vi "z2.vi"() -> ()   [LabVIEW 2023]
uses:
  Kontrola.ctl
panel:
  in  "10D":bool
  in  "5D":bool
  in  "stop 2":bool
  out "Numeric 3":dbl
  in  "stop":bool
  out "Numeric 2":dbl
  in  "Broj2":dbl
  in  "Broj 1":dbl
  in  "Dijeljenje":bool
  in  "Mnozenje":bool
  in  "Oduzimanje":bool
  in  "Sabiranje":bool
  in  "Numeric":i64
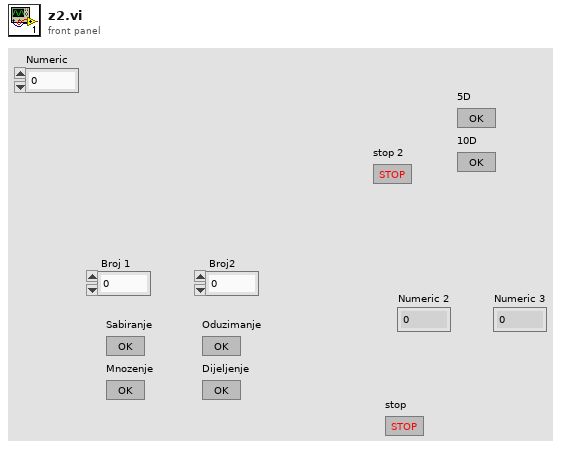
[diagram p1: front panel]
types:
  T1 = typedef "Kontrola.ctl" = enum16{"Init", "Shutdown", "5D", "10D", "15D", "20D", "Kusur"}
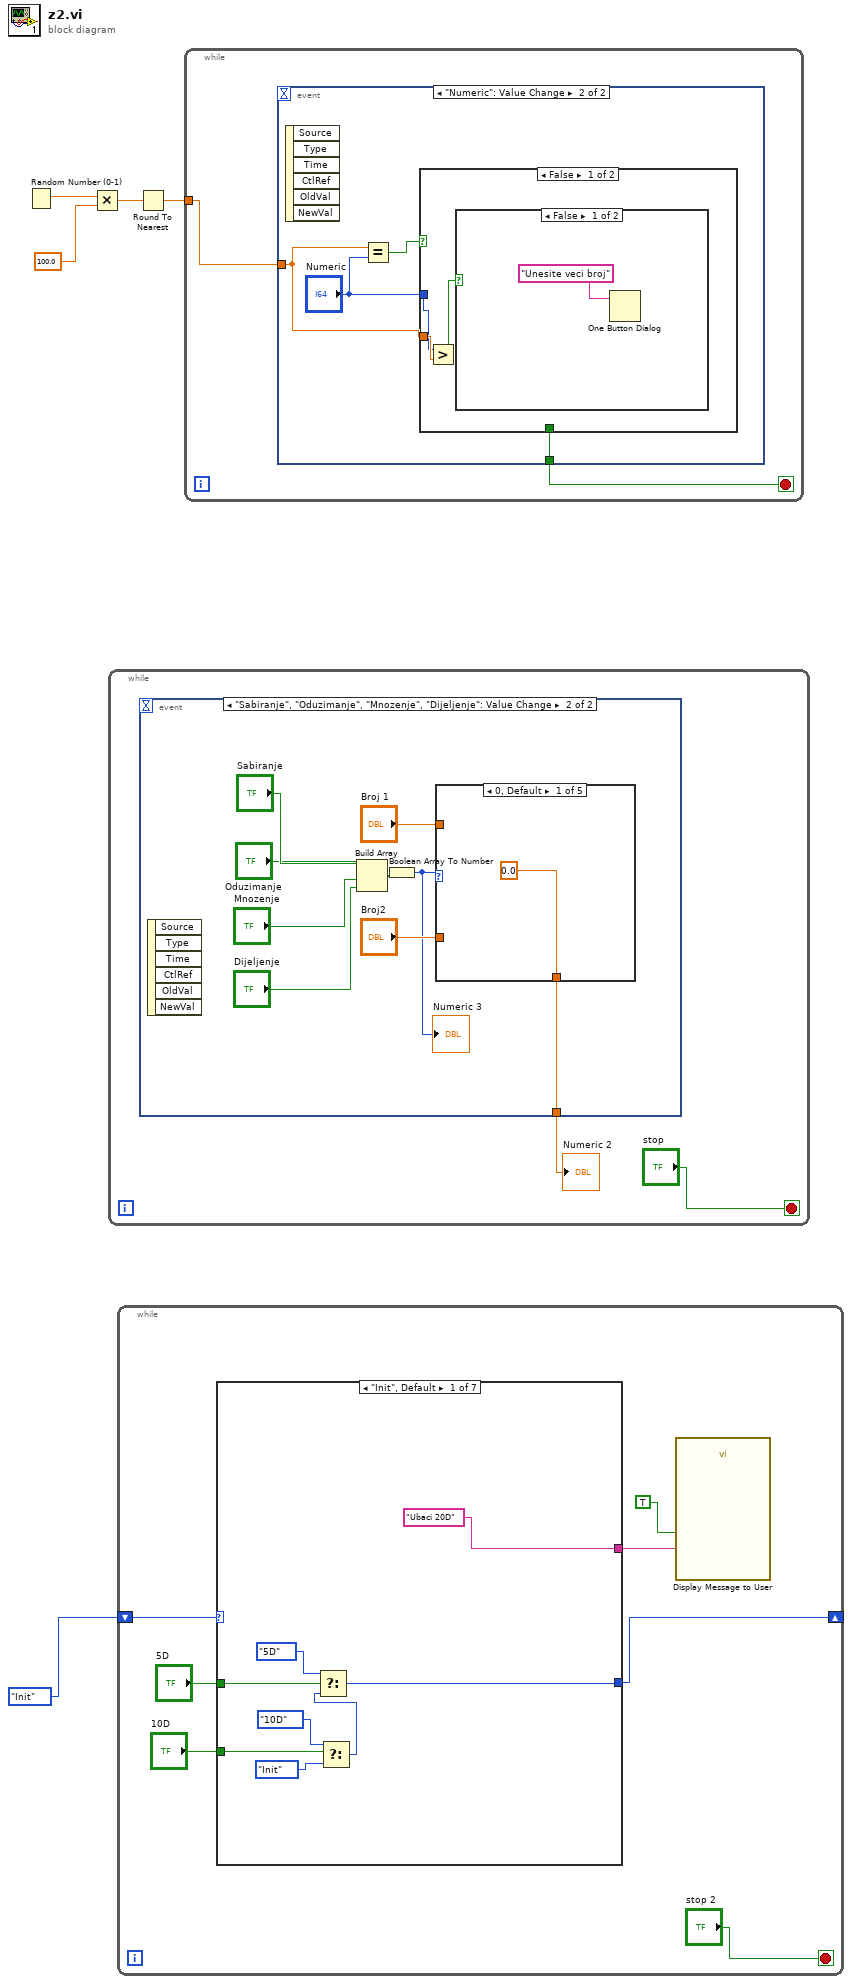
[diagram p0: block diagram]
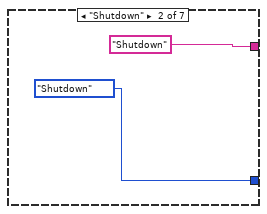
[diagram p2: hidden frame]
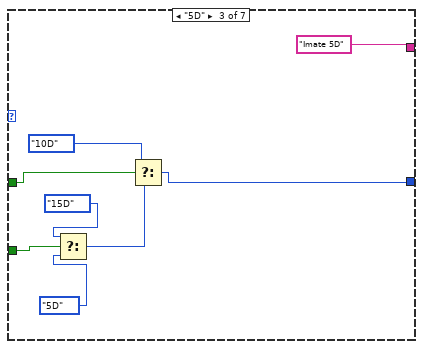
[diagram p3: hidden frame]
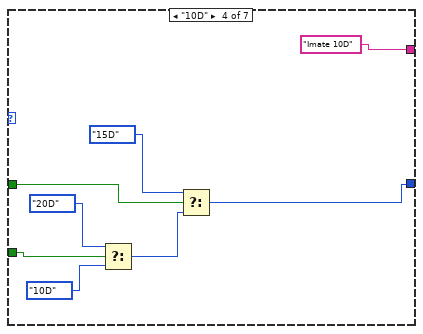
[diagram p4: hidden frame]
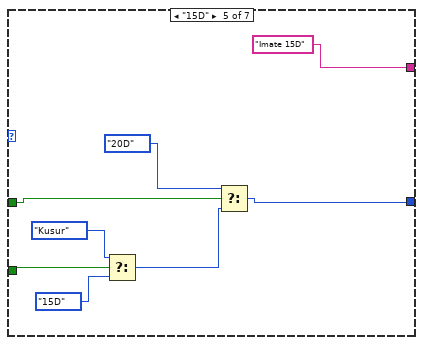
[diagram p5: hidden frame]
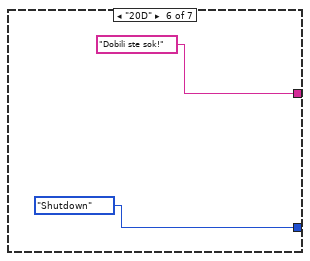
[diagram p6: hidden frame]
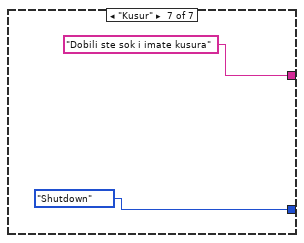
[diagram p7: hidden frame]
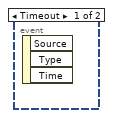
[diagram p8: hidden frame]
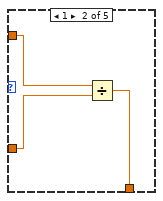
[diagram p9: hidden frame]
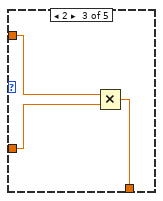
[diagram p10: hidden frame]
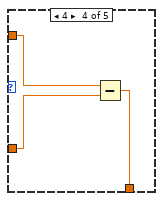
[diagram p11: hidden frame]
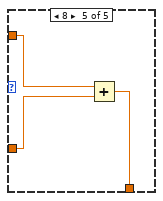
[diagram p12: hidden frame]
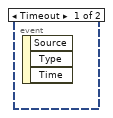
[diagram p13: hidden frame]
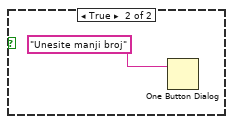
[diagram p14: hidden frame]
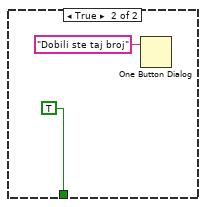
[diagram p15: hidden frame]
diagram:
  n1 = Random Number (0-1)() -> (number: 0 to 1=w4:dbl)
  n2 = Multiply(x=w4, y=100.0) -> (x*y=w3:dbl)
  n3 = while {
    stop <- "stop" stop-if-true
    n4 = event shown="[1] \"Sabiranje\", \"Oduzimanje\", \"Mnozenje\", \"Dijeljenje\": Value Change" {
      selector: _ -> [_ _]
      dyn-events: _ -> [_ _]
      timeout: _ -> [_ _]
      tunnel: [_ w11] -> w7
      event Timeout {
        n5 = event-data() -> ()  [unwired: 1 in, 3 out]
      }
      event "Sabiranje", "Oduzimanje", "Mnozenje", "Dijeljenje": Value Change {
        n6 = event-data() -> ()  [unwired: 1 in, 6 out]
        n7 = Build Array("Sabiranje", "Oduzimanje", "Mnozenje", "Dijeljenje") -> (w12:bool[])
        n8 = Boolean Array To Number(Boolean array=w12) -> (number=w8:u32)
        "Numeric 3" <- w8
        n9 = case shown="0, Default" w8 {
          tunnel: [0.0 w18 w21 w26 w27] -> w11
          tunnel: "Broj 1" -> [_ w20 w23 w25 w29]
          tunnel: "Broj2" -> [_ w19 w22 w24 w28]
          frame 0, Default {
          }
          frame 1 {
            n10 = Divide(x=w20, y=w19) -> (x/y=w18:dbl)
          }
          frame 2 {
            n11 = Multiply(x=w23, y=w22) -> (x*y=w21:dbl)
          }
          frame 4 {
            n12 = Subtract(x=w25, y=w24) -> (x-y=w26:dbl)
          }
          frame 8 {
            n13 = Add(x=w29, y=w28) -> (x+y=w27:dbl)
          }
        }
      }
    }
    "Numeric 2" <- w7
  }
  n14 = while {
    shift-right: [w32] -> _
    shift-left: Kontrola."Init" ("Enum") -> [w35]
    stop <- "stop 2" stop-if-true
    n15 = case shown="\"Init\", Default" w35 {
      tunnel: "5D" -> [w41 _ w54 w62 w70 _ _]
      tunnel: "10D" -> [w40 _ w52 w58 w68 _ _]
      tunnel: [w38 Kontrola."Shutdown" ("Enum") w48 w56 w64 Kontrola."Shutdown" ("Enum") Kontrola."Shutdown" ("Enum")] -> w32
      tunnel: ["Ubaci 20D" "Shutdown" "Imate 5D" "Imate 10D" "Imate 15D" "Dobili ste sok!" "Dobili ste sok i imate kusura"] -> w30
      frame "Init", Default {
        n16 = Select(t=Kontrola."10D" ("Enum"), s=w40, f=Kontrola."Init" ("Enum")) -> (s? t:f=w42:T1)
        n17 = Select(t=Kontrola."5D" ("Enum"), s=w41, f=w42) -> (s? t:f=w38:T1)
      }
      frame "Shutdown" {
      }
      frame "5D" {
        n18 = Select(t=Kontrola."15D" ("Enum"), s=w52, f=Kontrola."5D" ("Enum")) -> (s? t:f=w53:T1)
        n19 = Select(t=Kontrola."10D" ("Enum"), s=w54, f=w53) -> (s? t:f=w48:T1)
      }
      frame "10D" {
        n20 = Select(t=Kontrola."20D" ("Enum"), s=w58, f=Kontrola."10D" ("Enum")) -> (s? t:f=w61:T1)
        n21 = Select(t=Kontrola."15D" ("Enum"), s=w62, f=w61) -> (s? t:f=w56:T1)
      }
      frame "15D" {
        n22 = Select(t=Kontrola."Kusur" ("Enum"), s=w68, f=Kontrola."15D" ("Enum")) -> (s? t:f=w69:T1)
        n23 = Select(t=Kontrola."20D" ("Enum"), s=w70, f=w69) -> (s? t:f=w64:T1)
      }
      frame "20D" {
      }
      frame "Kusur" {
      }
    }
    n24 = call "Display Message to User"("Enable"=TRUE, "Message"=w30) -> ()  [unwired: 8 in, 2 out]
  }
  n25 = Round To Nearest(number=w3) -> (nearest integer value=w2:dbl)
  n26 = while {
    tunnel: w2 -> [w76]
    stop <- w75 stop-if-true
    n27 = event shown="[1] \"Numeric\": Value Change" {
      selector: _ -> [_ _]
      dyn-events: _ -> [_ _]
      timeout: _ -> [_ _]
      tunnel: w76 -> [_ w79]
      tunnel: [_ w77] -> w75
      event Timeout {
        n28 = event-data() -> ()  [unwired: 1 in, 3 out]
      }
      event "Numeric": Value Change {
        n29 = event-data() -> ()  [unwired: 1 in, 6 out]
        n30 = Equal?(x=w79, y="Numeric") -> (x = y?=w80:bool)
        n31 = case shown="False" w80 {
          tunnel: w79 -> [w83 _]
          tunnel: "Numeric" -> [w82 _]
          tunnel: [_ TRUE] -> w77
          frame False {
            n32 = Greater?(x=w82, y=w83) -> (0:w81:bool)
            n33 = case shown="False" w81 {
              frame False {
                n34 = One Button Dialog(message="Unesite veci broj") -> ()  [unwired: 1 in, 1 out]
              }
              frame True {
                n35 = One Button Dialog(message="Unesite manji broj") -> ()  [unwired: 1 in, 1 out]
              }
            }
          }
          frame True {
            n36 = One Button Dialog(message="Dobili ste taj broj") -> ()  [unwired: 1 in, 1 out]
          }
        }
      }
    }
  }
